vi "Create All Message Queues.vi"(8 "error in (no error)":errorcluster) -> (0 "error out":errorcluster, 3 "Message Queues out":T1)   [LabVIEW 2014, in "Message Queue.lvlib"]
doc: "This VI creates and initializes all the message queues for your application. If your application requires more than one message queue, right-click the \"Message Queues\" constant above and select Open Type Def. Add the new Message Queue(s) to the type definition, then initialize them in this VI."
uses:
  Message Queue.lvlib
  All Message Queues.ctl
  Message Cluster.ctl
  Digital/Digital Input Cluster.ctl
  Digital/Digital Output Cluster.ctl
  Data Processor/Data Processor cluster.ctl
  Data Processor/I Adj Parameters.ctl
  Laser/Keyence data cluster.ctl
  Laser/Keyence Status.ctl
  Analog/Analog Output Cluster.ctl
  UI/UI data.ctl
  Enqueue Message (Single).vi
  Lossy Enqueue Message (Single).vi
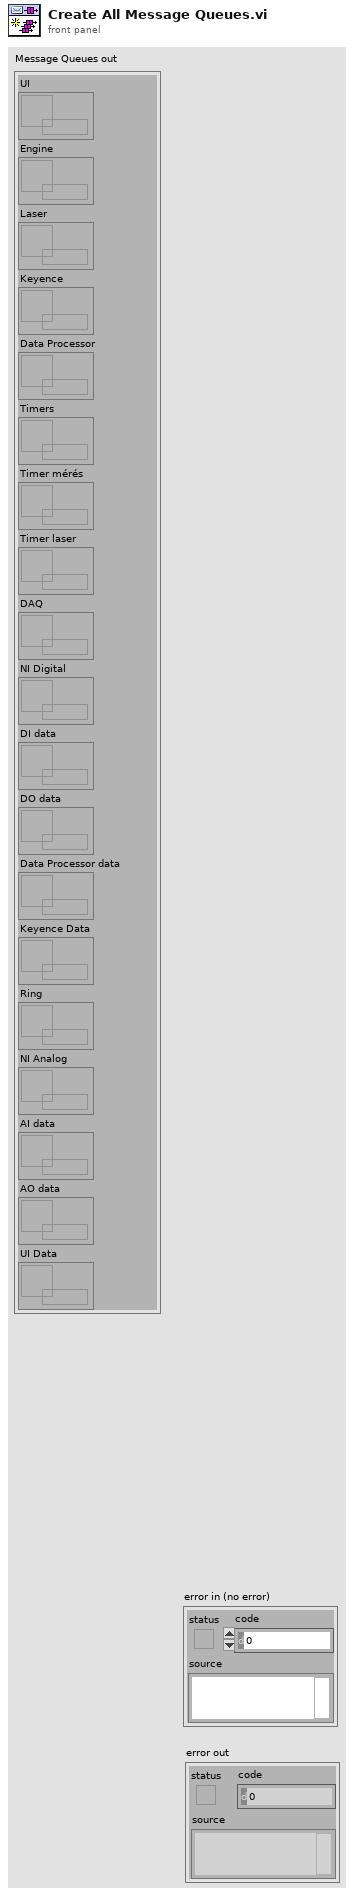
[diagram p1: front panel]
types:
  T1 = typedef "Message Queue.lvlib/All Message Queues.ctl" = cluster{"UI":refnum<queue>, "Engine":refnum<queue>, "Laser":refnum<queue>, "Keyence":refnum<queue>, "Data Processor":refnum<queue>, "Timers":refnum<queue>, "Timer mérés":refnum<queue>, "Timer laser":refnum<queue>, "DAQ":refnum<queue>, "NI Digital":refnum<queue>, "DI data":refnum<queue>, "DO data":refnum<queue>, "Data Processor data":refnum<queue>, "Keyence Data":refnum<queue>, "Ring":refnum<queue>, "NI Analog":refnum<queue>, "AI data":refnum<queue>, "AO data":refnum<queue>, "UI Data":refnum<queue>}
  T2 = typedef "Digital Input Cluster.ctl" = cluster{"PCIE-6321 IN":cluster{"Termék bördelezve":bool, "Izolációs relék OK":bool, "Rézgyûrû a terméken":bool, "Termék rögzítve":bool, "Termék a gyûrûzõben":bool, "Rézgyûrû behelyezve":bool, "Rézgyûrû elengedve":bool, "Rézgyûrû megnyomva":bool, "Termék elengedve":bool, "Levegõ rendben":bool, "Termék jelen (táv)":bool, "Termék jelen (fém)":bool, "Selejt érzékelõ":bool}}
  T3 = typedef "Digital Output Cluster.ctl" = cluster{"PCIE-6321 OUT":cluster{"Izolációs relé":bool, "B oldal relé (nincs használva)":bool, "48V relé":bool, "Elszívás KI":bool, "Bördelezés teszt":bool, "Gyûrû megnyomás":bool, "Termék rögzítés":bool, "R mérés relé":bool, "200mA relé":bool, "NTC mérés relé":bool, "Levegõ BE":bool}}
  T4 = typedef "Data Processor cluster.ctl" = cluster{"Dummy":bool, "R Res":dbl, "NTC Res":dbl, "Insulation Res":dbl, "Temperature":dbl, "NTC Exp Res":dbl, "NTC Calc Temp":dbl, "Delta U Puffer":refnum<queue>, "I Adj Parameters":T5, "UCTRL Cluster":cluster{"UCTRL NTC":dbl, "UCTRL R":dbl, "UCTRL dU":dbl}}
  T5 = typedef "I Adj Parameters.ctl" = cluster{"Vr NTC":dbl, "Vr R":dbl, "Vr dU":dbl, "I Adj step":i32, "Output":dbl, "Adj Failed":bool}
  T6 = typedef "Keyence data cluster.ctl" = cluster{"Communication Opened":bool, "Status":T7, "IP Address":string, "Laser Disabled":bool}
  T7 = typedef "Keyence Status.ctl" = cluster{"Ready":bool, "Error":bool, "Warning":bool, "Shutter":bool, "Mark Check OK":bool, "Mark Check NG":bool, "Marking Busy":bool, "Program No":u16, "Marking Check Busy":bool, "Marking Completed":bool, "Marking Score":u16, "Marking Error":bool, "Marking Stop":bool, "Program is changing":bool, "Date/Time":timestamp}
  T8 = typedef "Analog Output Cluster.ctl" = cluster{"NI-6221":cluster{"UCTRL":dbl}}
  T9 = typedef "UI data.ctl" = cluster{"AI engedélyezés":bool}
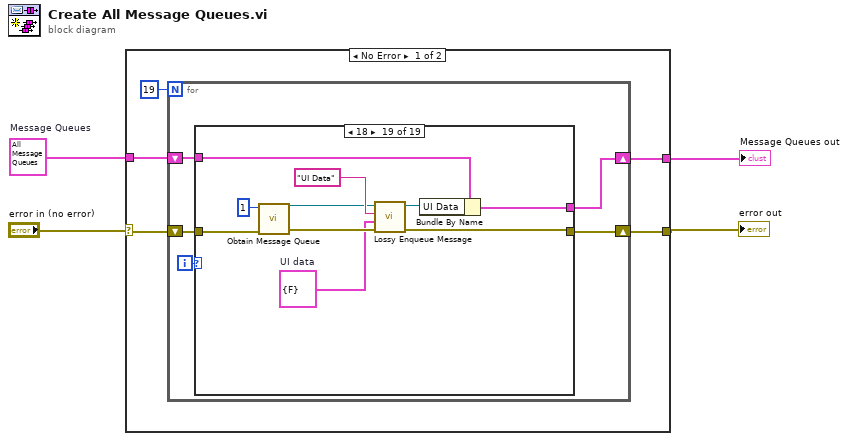
[diagram p0: block diagram]
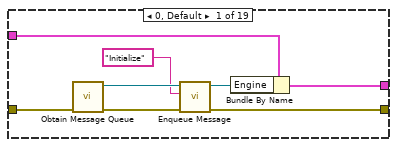
[diagram p2: hidden frame]
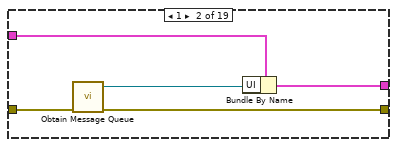
[diagram p3: hidden frame]
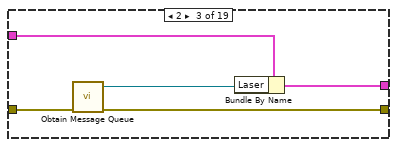
[diagram p4: hidden frame]
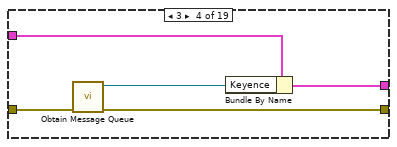
[diagram p5: hidden frame]
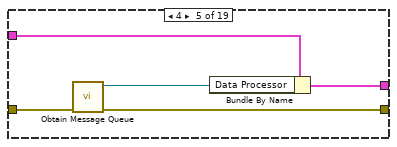
[diagram p6: hidden frame]
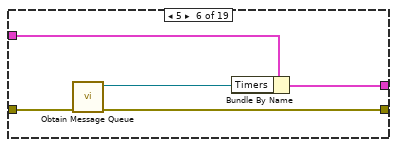
[diagram p7: hidden frame]
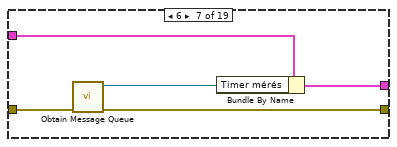
[diagram p8: hidden frame]
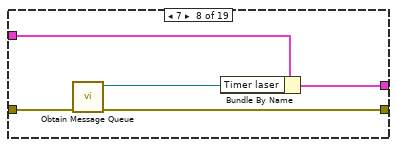
[diagram p9: hidden frame]
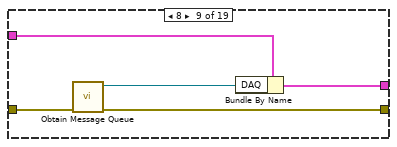
[diagram p10: hidden frame]
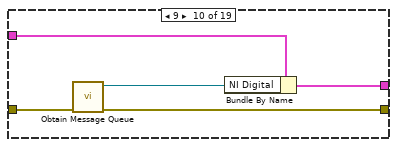
[diagram p11: hidden frame]
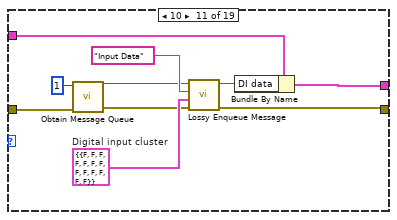
[diagram p12: hidden frame]
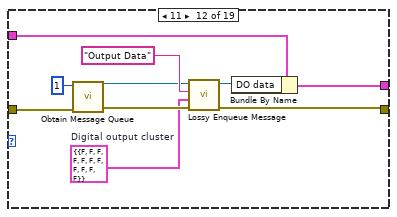
[diagram p13: hidden frame]
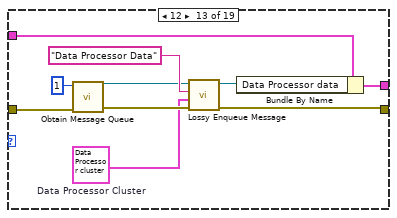
[diagram p14: hidden frame]
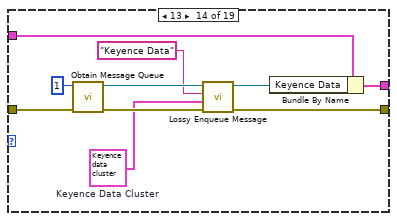
[diagram p15: hidden frame]
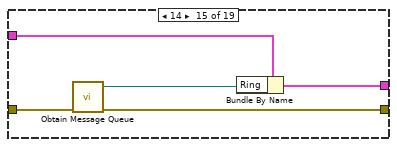
[diagram p16: hidden frame]
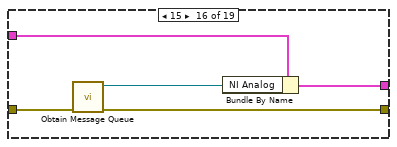
[diagram p17: hidden frame]
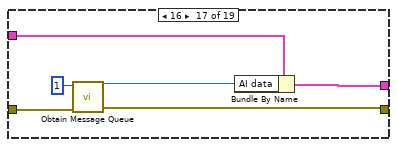
[diagram p18: hidden frame]
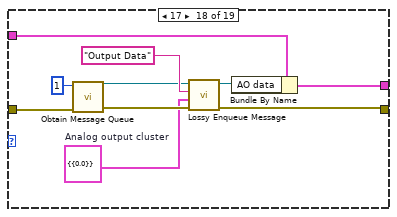
[diagram p19: hidden frame]
diagram:
  w3 = T1 {"UI"=refnum, "Engine"=refnum, "Laser"=refnum, "Keyence"=refnum, "Data Processor"=refnum, "Timers"=refnum, "Timer mérés"=refnum, "Timer laser"=refnum, "DAQ"=refnum, "NI Digital"=refnum, "DI data"=refnum, "DO data"=refnum, "Data Processor data"=refnum, "Keyence Data"=refnum, "Ring"=refnum, "NI Analog"=refnum, "AI data"=refnum, "AO data"=refnum, "UI Data"=refnum}  # Message Queues
  n1 = case shown="No Error" "error in (no error)" {
    selector: "error in (no error)" -> [w9 w145]
    tunnel: w3 -> [w8 w144]
    tunnel: [w6 w144] -> w2
    tunnel: [w5 w145] -> w1
    frame No Error {
      n2 = for {
        N: 19 -> [_]
        shift-right: [w12] -> w5
        shift-left: w9 -> [w11]
        shift-right: [w14] -> w6
        shift-left: w8 -> [w13]
        i -> [w10]
        n3 = case shown="18" w10 {
          tunnel: w11 -> [w20 w25 w30 w34 w39 w44 w49 w54 w59 w64 w75 w85 w95 w105 w110 w114 w121 w131 w141]
          tunnel: w13 -> [w22 w27 w32 w37 w42 w47 w52 w57 w62 w67 w77 w87 w97 w107 w112 w117 w123 w133 w143]
          tunnel: [w21 w26 w31 w36 w41 w46 w51 w56 w61 w66 w76 w86 w96 w106 w111 w116 w122 w132 w142] -> w14
          tunnel: [w15 w24 w29 w33 w38 w43 w48 w53 w58 w63 w68 w79 w89 w100 w109 w113 w118 w125 w135] -> w12
          frame 0, Default {
            n4 = call "Obtain Message Queue.vi"("error in (no error)"=w20) -> ("error out"=w19:errorcluster, "Message Queue"=w18:refnum<queue>)  [unwired: 9 in]
            n5 = call-poly "Enqueue Message.vi"("error in (no error)"=w19, "Message"="Initialize", "Message Queue"=w18) -> ("error out"=w15:errorcluster, "dup Message Queue"=w17:refnum<queue>)  [unwired: 7 in]
            n6 = Bundle By Name(cluster=w22, "Engine"=w17) -> (w21:T1)
          }
          frame 1 {
            n7 = call "Obtain Message Queue.vi"("error in (no error)"=w25) -> ("error out"=w24:errorcluster, "Message Queue"=w23:refnum<queue>)  [unwired: 9 in]
            n8 = Bundle By Name(cluster=w27, "UI"=w23) -> (w26:T1)
          }
          frame 2 {
            n9 = call "Obtain Message Queue.vi"("error in (no error)"=w30) -> ("error out"=w29:errorcluster, "Message Queue"=w28:refnum<queue>)  [unwired: 9 in]
            n10 = Bundle By Name(cluster=w32, "Laser"=w28) -> (w31:T1)
          }
          frame 3 {
            n11 = call "Obtain Message Queue.vi"("error in (no error)"=w34) -> ("error out"=w33:errorcluster, "Message Queue"=w35:refnum<queue>)  [unwired: 9 in]
            n12 = Bundle By Name(cluster=w37, "Keyence"=w35) -> (w36:T1)
          }
          frame 4 {
            n13 = call "Obtain Message Queue.vi"("error in (no error)"=w39) -> ("error out"=w38:errorcluster, "Message Queue"=w40:refnum<queue>)  [unwired: 9 in]
            n14 = Bundle By Name(cluster=w42, "Data Processor"=w40) -> (w41:T1)
          }
          frame 5 {
            n15 = call "Obtain Message Queue.vi"("error in (no error)"=w44) -> ("error out"=w43:errorcluster, "Message Queue"=w45:refnum<queue>)  [unwired: 9 in]
            n16 = Bundle By Name(cluster=w47, "Timers"=w45) -> (w46:T1)
          }
          frame 6 {
            n17 = call "Obtain Message Queue.vi"("error in (no error)"=w49) -> ("error out"=w48:errorcluster, "Message Queue"=w50:refnum<queue>)  [unwired: 9 in]
            n18 = Bundle By Name(cluster=w52, "Timer mérés"=w50) -> (w51:T1)
          }
          frame 7 {
            n19 = call "Obtain Message Queue.vi"("error in (no error)"=w54) -> ("error out"=w53:errorcluster, "Message Queue"=w55:refnum<queue>)  [unwired: 9 in]
            n20 = Bundle By Name(cluster=w57, "Timer laser"=w55) -> (w56:T1)
          }
          frame 8 {
            n21 = call "Obtain Message Queue.vi"("error in (no error)"=w59) -> ("error out"=w58:errorcluster, "Message Queue"=w60:refnum<queue>)  [unwired: 9 in]
            n22 = Bundle By Name(cluster=w62, "DAQ"=w60) -> (w61:T1)
          }
          frame 9 {
            n23 = call "Obtain Message Queue.vi"("error in (no error)"=w64) -> ("error out"=w63:errorcluster, "Message Queue"=w65:refnum<queue>)  [unwired: 9 in]
            n24 = Bundle By Name(cluster=w67, "NI Digital"=w65) -> (w66:T1)
          }
          frame 10 {
            w70 = T2 {"PCIE-6321 IN"={"Termék bördelezve"=FALSE, "Izolációs relék OK"=FALSE, "Rézgyûrû a terméken"=FALSE, "Termék rögzítve"=FALSE, "Termék a gyûrûzõben"=FALSE, "Rézgyûrû behelyezve"=FALSE, "Rézgyûrû elengedve"=FALSE, "Rézgyûrû megnyomva"=FALSE, "Termék elengedve"=FALSE, "Levegõ rendben"=FALSE, "Termék jelen (táv)"=FALSE, "Termék jelen (fém)"=FALSE, "Selejt érzékelõ"=FALSE}}  # Digital input cluster
            n25 = call "Obtain Message Queue.vi"("error in (no error)"=w75, "max queue size (-1, unlimited)"=1) -> ("error out"=w69:errorcluster, "Message Queue"=w71:refnum<queue>)  [unwired: 8 in]
            n26 = call-poly "Lossy Enqueue Message.vi"("error in (no error)"=w69, "Message Data"=w70, "Message"="Input Data", "Message Queue"=w71) -> ("error out"=w68:errorcluster, "dup Message Queue"=w72:refnum<queue>)  [unwired: 6 in]
            n27 = Bundle By Name(cluster=w77, "DI data"=w72) -> (w76:T1)
          }
          frame 11 {
            w78 = T3 {"PCIE-6321 OUT"={"Izolációs relé"=FALSE, "B oldal relé (nincs használva)"=FALSE, "48V relé"=FALSE, "Elszívás KI"=FALSE, "Bördelezés teszt"=FALSE, "Gyûrû megnyomás"=FALSE, "Termék rögzítés"=FALSE, "R mérés relé"=FALSE, "200mA relé"=FALSE, "NTC mérés relé"=FALSE, "Levegõ BE"=FALSE}}  # Digital output cluster
            n28 = call "Obtain Message Queue.vi"("error in (no error)"=w85, "max queue size (-1, unlimited)"=1) -> ("error out"=w80:errorcluster, "Message Queue"=w81:refnum<queue>)  [unwired: 8 in]
            n29 = call-poly "Lossy Enqueue Message.vi"("error in (no error)"=w80, "Message Data"=w78, "Message"="Output Data", "Message Queue"=w81) -> ("error out"=w79:errorcluster, "dup Message Queue"=w82:refnum<queue>)  [unwired: 6 in]
            n30 = Bundle By Name(cluster=w87, "DO data"=w82) -> (w86:T1)
          }
          frame 12 {
            w88 = T4 {"Dummy"=FALSE, "R Res"=0.0, "NTC Res"=0.0, "Insulation Res"=0.0, "Temperature"=0.0, "NTC Exp Res"=0.0, "NTC Calc Temp"=0.0, "Delta U Puffer"=refnum, "I Adj Parameters"={"Vr NTC"=0.0, "Vr R"=0.0, "Vr dU"=0.0, "I Adj step"=0, "Output"=0.0, "Adj Failed"=FALSE}, "UCTRL Cluster"={"UCTRL NTC"=0.0, "UCTRL R"=0.0, "UCTRL dU"=0.0}}  # Data Processor Cluster
            n31 = call "Obtain Message Queue.vi"("error in (no error)"=w95, "max queue size (-1, unlimited)"=1) -> ("error out"=w90:errorcluster, "Message Queue"=w91:refnum<queue>)  [unwired: 8 in]
            n32 = call-poly "Lossy Enqueue Message.vi"("error in (no error)"=w90, "Message Data"=w88, "Message"="Data Processor Data", "Message Queue"=w91) -> ("error out"=w89:errorcluster, "dup Message Queue"=w92:refnum<queue>)  [unwired: 6 in]
            n33 = Bundle By Name(cluster=w97, "Data Processor data"=w92) -> (w96:T1)
          }
          frame 13 {
            w99 = T6 {"Communication Opened"=FALSE, "Status"={"Ready"=FALSE, "Error"=FALSE, "Warning"=FALSE, "Shutter"=FALSE, "Mark Check OK"=FALSE, "Mark Check NG"=FALSE, "Marking Busy"=FALSE, "Program No"=0, "Marking Check Busy"=FALSE, "Marking Completed"=FALSE, "Marking Score"=0, "Marking Error"=FALSE, "Marking Stop"=FALSE, "Program is changing"=FALSE, "Date/Time"=timestamp(0 s since 1904-01-01)}, "IP Address"="", "Laser Disabled"=FALSE}  # Keyence Data Cluster
            n34 = call "Obtain Message Queue.vi"("error in (no error)"=w105, "max queue size (-1, unlimited)"=1) -> ("error out"=w101:errorcluster, "Message Queue"=w103:refnum<queue>)  [unwired: 8 in]
            n35 = call-poly "Lossy Enqueue Message.vi"("error in (no error)"=w101, "Message Data"=w99, "Message"="Keyence Data", "Message Queue"=w103) -> ("error out"=w100:errorcluster, "dup Message Queue"=w102:refnum<queue>)  [unwired: 6 in]
            n36 = Bundle By Name(cluster=w107, "Keyence Data"=w102) -> (w106:T1)
          }
          frame 14 {
            n37 = call "Obtain Message Queue.vi"("error in (no error)"=w110) -> ("error out"=w109:errorcluster, "Message Queue"=w108:refnum<queue>)  [unwired: 9 in]
            n38 = Bundle By Name(cluster=w112, "Ring"=w108) -> (w111:T1)
          }
          frame 15 {
            n39 = call "Obtain Message Queue.vi"("error in (no error)"=w114) -> ("error out"=w113:errorcluster, "Message Queue"=w115:refnum<queue>)  [unwired: 9 in]
            n40 = Bundle By Name(cluster=w117, "NI Analog"=w115) -> (w116:T1)
          }
          frame 16 {
            n41 = call "Obtain Message Queue.vi"("error in (no error)"=w121, "max queue size (-1, unlimited)"=1) -> ("error out"=w118:errorcluster, "Message Queue"=w119:refnum<queue>)  [unwired: 8 in]
            n42 = Bundle By Name(cluster=w123, "AI data"=w119) -> (w122:T1)
          }
          frame 17 {
            w124 = T8 {"NI-6221"={"UCTRL"=0.0}}  # Analog output cluster
            n43 = call "Obtain Message Queue.vi"("error in (no error)"=w131, "max queue size (-1, unlimited)"=1) -> ("error out"=w126:errorcluster, "Message Queue"=w127:refnum<queue>)  [unwired: 8 in]
            n44 = call-poly "Lossy Enqueue Message.vi"("error in (no error)"=w126, "Message Data"=w124, "Message"="Output Data", "Message Queue"=w127) -> ("error out"=w125:errorcluster, "dup Message Queue"=w128:refnum<queue>)  [unwired: 6 in]
            n45 = Bundle By Name(cluster=w133, "AO data"=w128) -> (w132:T1)
          }
          frame 18 {
            w134 = T9 {"AI engedélyezés"=FALSE}  # UI data
            n46 = call "Obtain Message Queue.vi"("error in (no error)"=w141, "max queue size (-1, unlimited)"=1) -> ("error out"=w136:errorcluster, "Message Queue"=w137:refnum<queue>)  [unwired: 8 in]
            n47 = call-poly "Lossy Enqueue Message.vi"("error in (no error)"=w136, "Message Data"=w134, "Message"="UI Data", "Message Queue"=w137) -> ("error out"=w135:errorcluster, "dup Message Queue"=w138:refnum<queue>)  [unwired: 6 in]
            n48 = Bundle By Name(cluster=w143, "UI Data"=w138) -> (w142:T1)
          }
        }
      }
    }
    frame Error {
    }
  }
  "Message Queues out" <- w2
  "error out" <- w1
